vi "ADO Recordset Cache Size.vi"(0 "ADODB._Recordset In":refnum<k7>, 1 "CacheSize":i32, 5 "error in (no error)":errorcluster) -> (14 "ADODB._Recordset Out":refnum<k7>, 19 "error out":errorcluster)   [LabVIEW 2013]
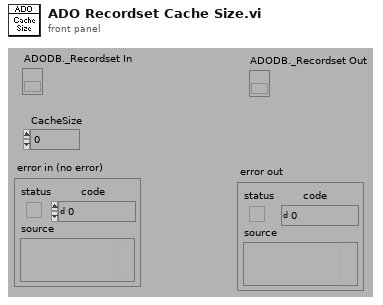
[diagram p1: front panel]
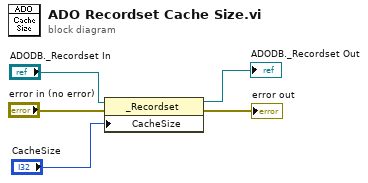
[diagram p0: block diagram]
diagram:
  n1 = property class="_Recordset"(reference="ADODB._Recordset In", error in="error in (no error)", "CacheSize"="CacheSize") -> (reference out=→"ADODB._Recordset Out":refnum<k7>, error out=→"error out":errorcluster)
